vi "scanTimingLogger.vi"(5 "duty":u16 format="%016b", 7 "mode":enum16{"Write", "Read", "Flush"}(ring), 9 "time":dbl, 11 "name":string) -> (1 "16-scanMeans":dbl[](array[numeric]) caption="<-Average" format="%0_2p", 2 "times":dbl[][](array[numeric]) format="%0_2p")   [LabVIEW 2021]
uses:
  <vilib>/Analysis/baseanly.llb/Mean (DBL).vi
  <vilib>/Analysis/NI_AALBase.lvlib
panel:
  out "16-scanMax":dbl[](array[numeric]) caption="<-Max" format="%0_2p"
  in  "threhold(s)":dbl=1.0 format="%0_2p"
  out "rowSum":dbl[](array[numeric]) format="%_3p"
  in  "tableLength":i32=16
  out "row":i32
  out "timeRead":dbl
  out "names":string[](array[string])
  # "Note: While individual channel times are correct, showing this VI will slow down the Scan Table overall"
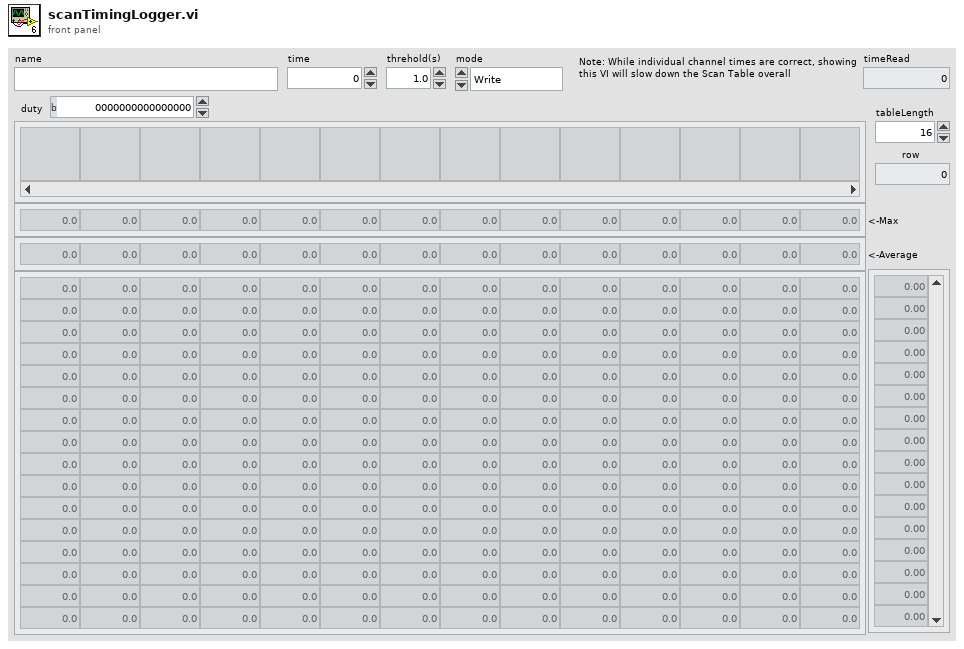
[diagram p1: front panel]
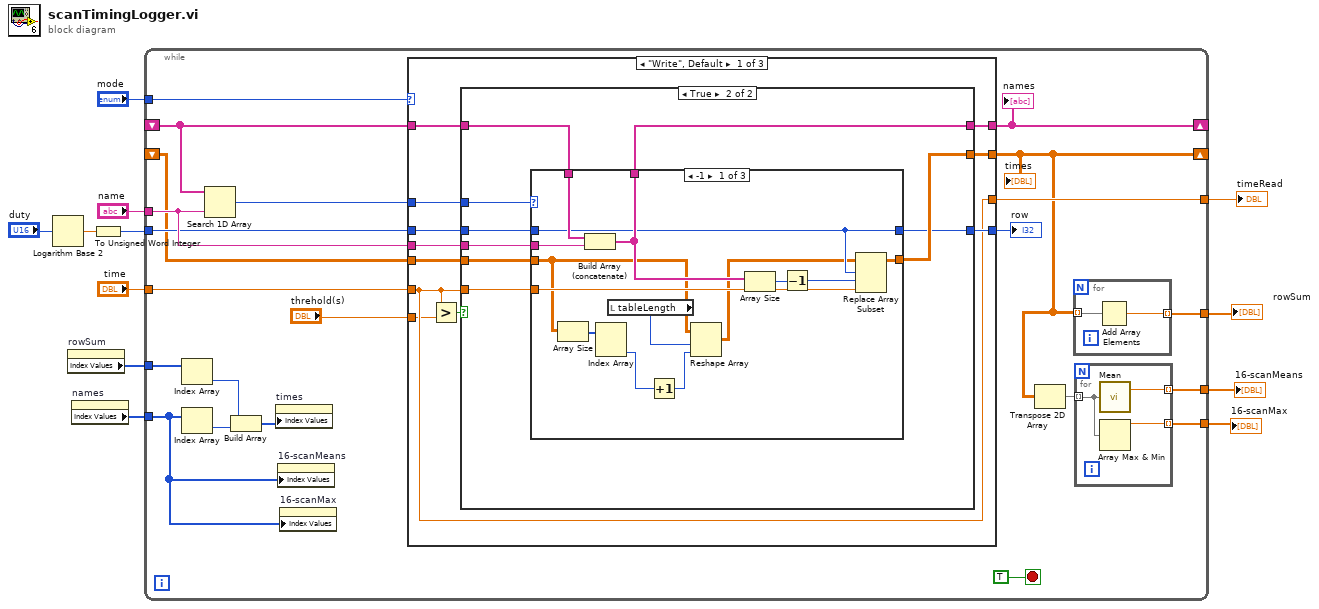
[diagram p0: block diagram]
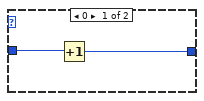
[diagram p3: hidden frame]
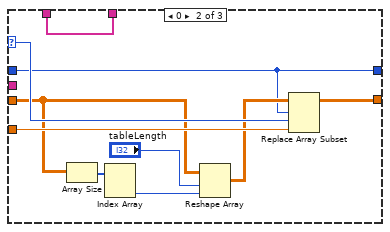
[diagram p4: hidden frame]
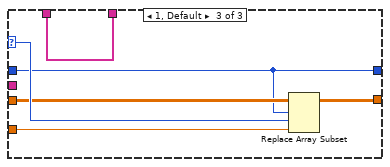
[diagram p5: hidden frame]
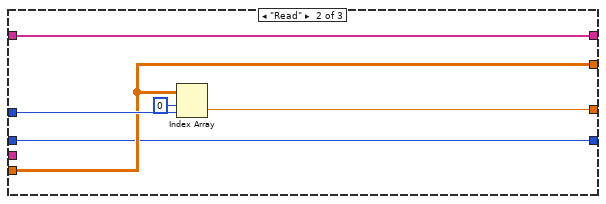
[diagram p6: hidden frame]
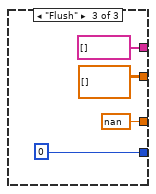
[diagram p7: hidden frame]
diagram:
  n1 = Logarithm Base 2(1:"duty") -> (0:w3:dbl)
  n2 = property on="rowSum" class="Arr (strict)"() -> ("Index Values"=w6:u32[])  [unwired: 2 in, 2 out]
  n3 = property on="names" class="Arr (strict)"() -> ("Index Values"=w8:u32[])  [unwired: 2 in, 2 out]
  n4 = To Unsigned Word Integer(number=w3) -> (unsigned 16bit integer=w2:u16)
  n5 = while {
    shift-right: [w27] -> _
    shift-left: _ -> [w32]
    shift-right: [w17] -> _
    shift-left: _ -> [w22]
    tunnel: "mode" -> [w33]
    tunnel: "name" -> [w31]
    tunnel: "time" -> [w30]
    tunnel: [w28] -> w9
    tunnel: w8 -> [w13]
    tunnel: w6 -> [w21]
    tunnel: [w19] -> w7
    tunnel: [w16] -> w5
    tunnel: w2 -> [w24]
    tunnel: [w14] -> w1
    stop <- TRUE stop-if-true
    n6 = Index Array(array=w21) -> (element=w20:u32)  [unwired: 1 in]
    n7 = Index Array(array=w13) -> (element=w25:u32)  [unwired: 1 in]
    n8 = Search 1D Array(1D array=w32, element=w31) -> (index of element=w29:i32)  [unwired: 1 in]
    n9 = Build Array(w20, w25) -> (w26:u32[])
    n10 = property on="times" class="Arr (strict)"("Index Values"=w26) -> ()  [unwired: 2 in, 2 out]
    n11 = property on="16-scanMeans" class="Arr (strict)"("Index Values"=w13) -> ()  [unwired: 2 in, 2 out]
    n12 = property on="16-scanMax" class="Arr (strict)"("Index Values"=w13) -> ()  [unwired: 2 in, 2 out]
    n13 = case shown="\"Write\", Default" w33 {
      tunnel: w32 -> [w48 w103 _]
      tunnel: [w49 w103 string[] [] ("names")] -> w27
      tunnel: w31 -> [w50 _ _]
      tunnel: [w45 w100 dbl[][] [] ("times")] -> w17
      tunnel: w30 -> [w42 _ _]
      tunnel: w29 -> [w47 w102 _]
      tunnel: [w42 w99 nan ("Numeric")] -> w28
      tunnel: w22 -> [w46 w100 _]
      tunnel: w24 -> [w44 w98 _]
      tunnel: [w43 w98 0] -> w23
      tunnel: "threhold(s)" -> [w40 _ _]
      frame "Write", Default {
        n14 = Greater?(x=w42, y=w40) -> (0:w41:bool)
        n15 = case shown="True" w41 {
          tunnel: w50 -> [_ w67]
          tunnel: [w55 w66] -> w49
          tunnel: w48 -> [w55 w65]
          tunnel: w47 -> [w53 w64]
          tunnel: w42 -> [_ w63]
          tunnel: w46 -> [w54 w62]
          tunnel: [w54 w61] -> w45
          tunnel: w44 -> [w52 w60]
          tunnel: [w51 w59] -> w43
          frame False {
            n16 = case shown="1, Default" w53 {
              tunnel: w52 -> [w57 w58]
              tunnel: [w56 w58] -> w51
              frame 0 {
                n17 = Increment(x=w57) -> (x+1=w56:u16)
              }
              frame 1, Default {
              }
            }
          }
          frame True {
            n18 = case shown="-1" w64 {
              selector: w64 -> [_ w90 w96]
              tunnel: w63 -> [w76 w91 w97]
              tunnel: [w78 w89 w95] -> w61
              tunnel: w65 -> [w81 w88 w94]
              tunnel: w67 -> [w80 _ _]
              tunnel: [w79 w88 w94] -> w66
              tunnel: w62 -> [w70 w84 w93]
              tunnel: w60 -> [w74 w83 w92]
              tunnel: [w74 w83 w92] -> w59
              frame -1 {
                n19 = Array Size(array=w70) -> (size(s)=w73:i32[])
                n20 = Build Array (concatenate)(w81, w80) -> (w79:string[])
                n21 = Index Array(array=w73) -> (element #2=w72:i32)  [unwired: 2 in, 1 out]
                n22 = local read "tableLength"() -> (w68:i32)
                n23 = Increment(x=w72) -> (x+1=w71:i32)
                n24 = Reshape Array(w70, w68, w71) -> (w69:dbl[][])
                n25 = Array Size(array=w79) -> (size(s)=w77:i32)
                n26 = Decrement(x=w77) -> (x-1=w75:i32)
                n27 = Replace Array Subset(array=w69, new element=w76, index (row)=w74, index (col)=w75) -> (w78:dbl[][])
              }
              frame 0 {
                n28 = Array Size(array=w84) -> (size(s)=w87:i32[])
                n29 = Index Array(array=w87) -> (element #2=w86:i32)  [unwired: 2 in, 1 out]
                n30 = Reshape Array(w84, "tableLength", w86) -> (w85:dbl[][])
                n31 = Replace Array Subset(array=w85, new element=w91, index (row)=w83, index (col)=w90) -> (w89:dbl[][])
              }
              frame 1, Default {
                n32 = Replace Array Subset(array=w93, new element=w97, index (row)=w92, index (col)=w96) -> (w95:dbl[][])
              }
            }
          }
        }
      }
      frame "Read" {
        n33 = Index Array(array=w100, index (row)=0 ("disabled index (row)"), index (col)=w102) -> (element=w99:dbl)
      }
      frame "Flush" {
      }
    }
    "names" <- w27
    "times" <- w17
    "row" <- w23
    n34 = Transpose 2D Array(2D array=w17) -> (transposed array=w18:dbl[][])
    n35 = for {
      tunnel: w17 -> [w39] mode=indexing
      tunnel: [w38] -> w19 mode=indexing
      n36 = Add Array Elements(numeric array=w39) -> (sum=w38:dbl)
    }
    n37 = for {
      tunnel: w18 -> [w36] mode=indexing
      tunnel: [w37] -> w16 mode=indexing
      tunnel: [w35] -> w14 mode=indexing
      n38 = call-poly <vilib>:"Mean.vi"("X"=w36) -> ("mean"=w37:dbl)  [unwired: 1 out]
      n39 = Array Max & Min(array=w36) -> (max value=w35:dbl)  [unwired: 3 out]
    }
  }
  "timeRead" <- w9
  "rowSum" <- w7
  "16-scanMeans" <- w5
  "16-scanMax" <- w1
